vi "FormProductsTable.vi"() -> ()   [LabVIEW 2012]
uses:
  resultShow.vi
  S7Ref.vi
panel:
  in  "判定设定 2":string[][](table)
  in  "参数设定 2":string[][](table)
  in  "判定设定":string[][](table)
  in  "参数设定":string[][](table)
  in  "功能选择":T1
  in  "产品选择":bool
  in  "产品删除":bool
  in  "产品更新":bool
  in  "产品注册":bool
  in  "产品":string(combo)
  # "磨合速度"
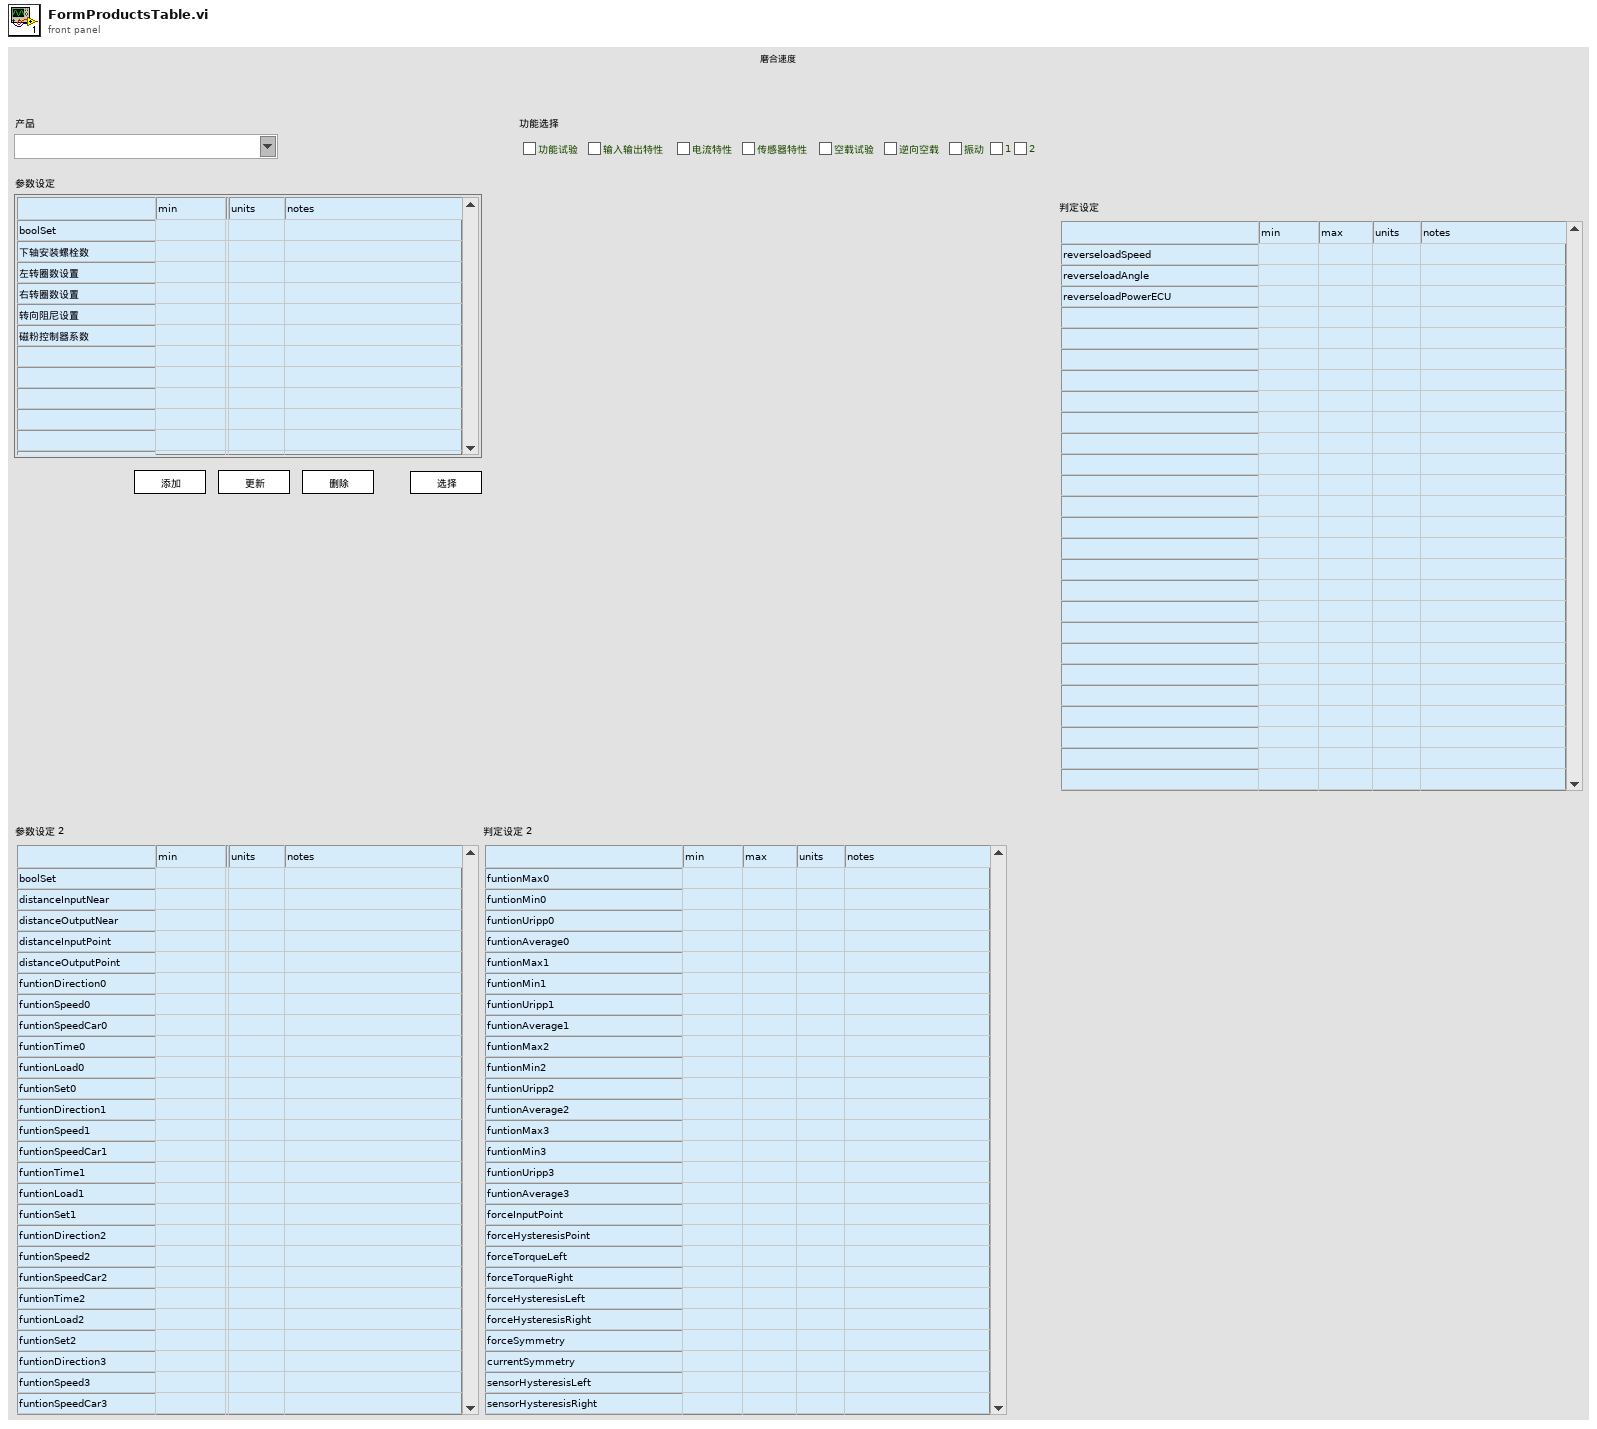
[diagram p1: front panel]
types:
  T1 = cluster{"功能试验":bool, "输入输出特性":bool, "电流特性":bool, "传感器特性":bool, "空载试验":bool, "逆向空载":bool, "振动":bool, "1":bool, "2":bool}
  T2 = enum8{"Enabled", "Disabled", "Disabled and Grayed Out"}
  T3 = enum16{"selectdata", "selectsave", "selectlist", "selectshow"}
  T4 = cluster{"userCode":string, "userName":string, "userStatus":string, "connectionMode":string, "takesTime":string, "countDone":string, "countOK":string, "countNG":string, "rigStatus":string, "productsName":string, "partCode1":string, "partCode2":string, "partCode3":string}
  T5 = cluster{"Boolean array[0]":bool, "Boolean array[1]":bool, "Boolean array[2]":bool, "Boolean array[3]":bool, "Boolean array[4]":bool, "Boolean array[5]":bool, "Boolean array[6]":bool, "Boolean array[7]":bool, "Boolean array[8]":bool}
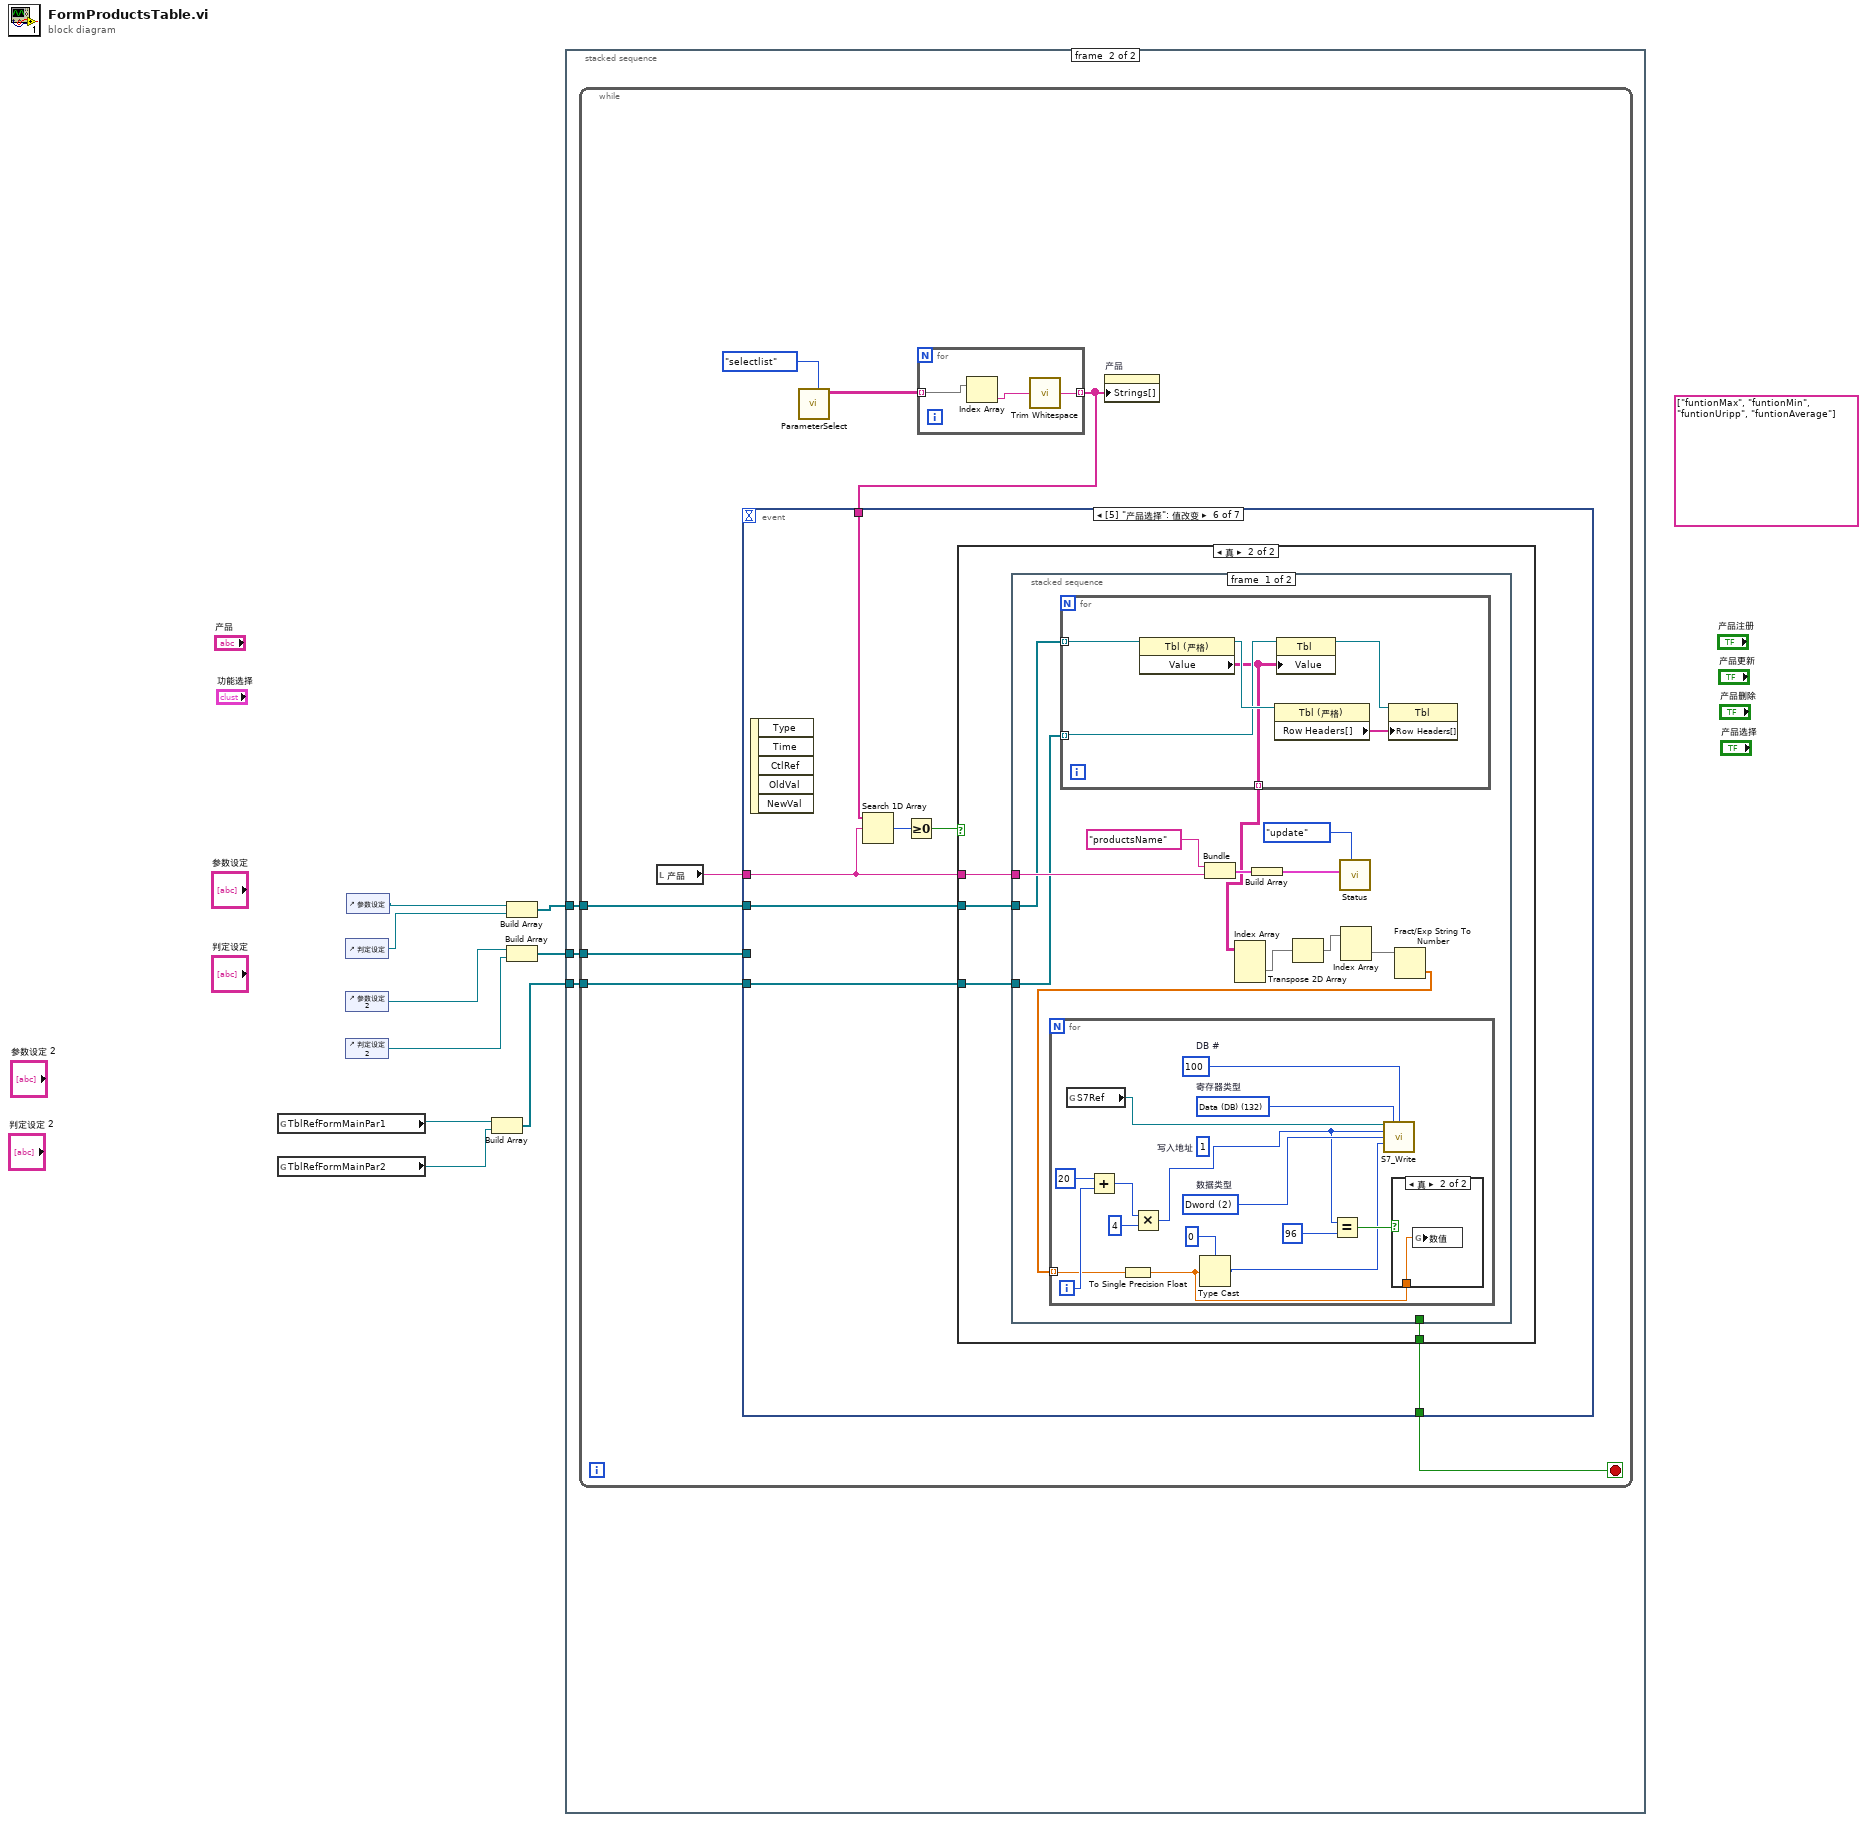
[diagram p0: block diagram]
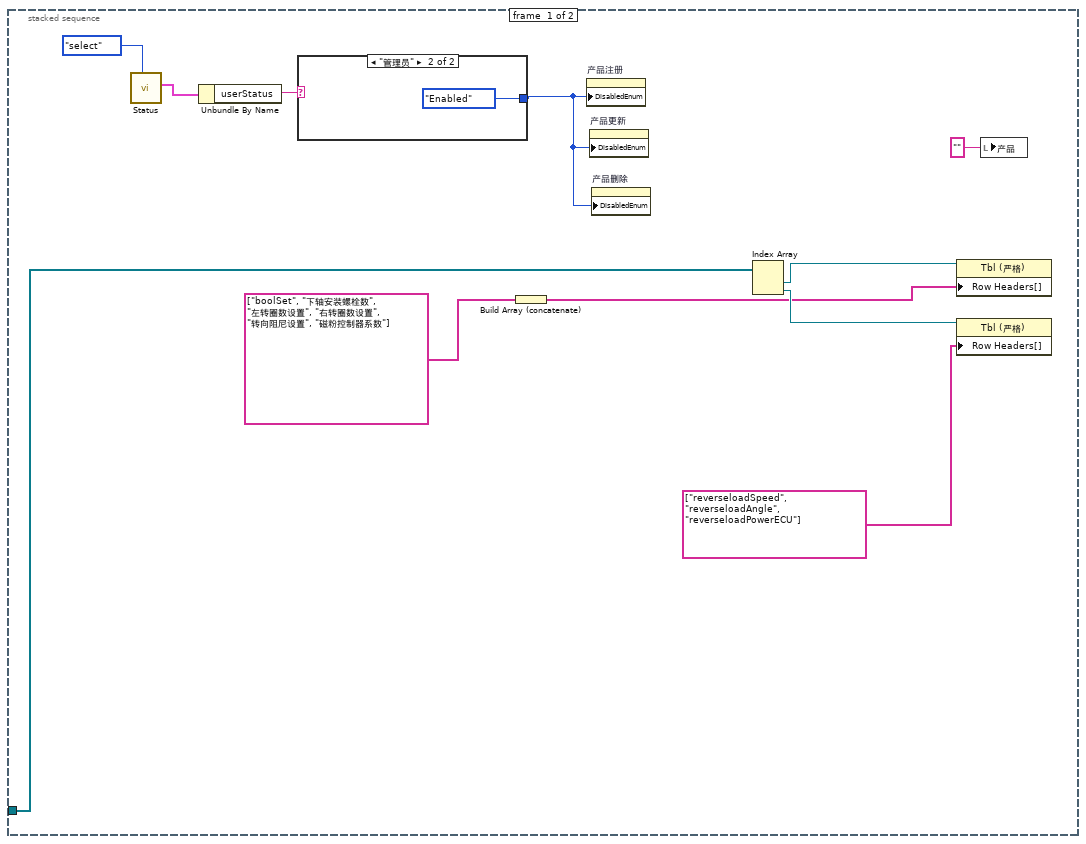
[diagram p2: hidden frame]
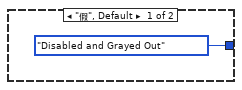
[diagram p3: hidden frame]
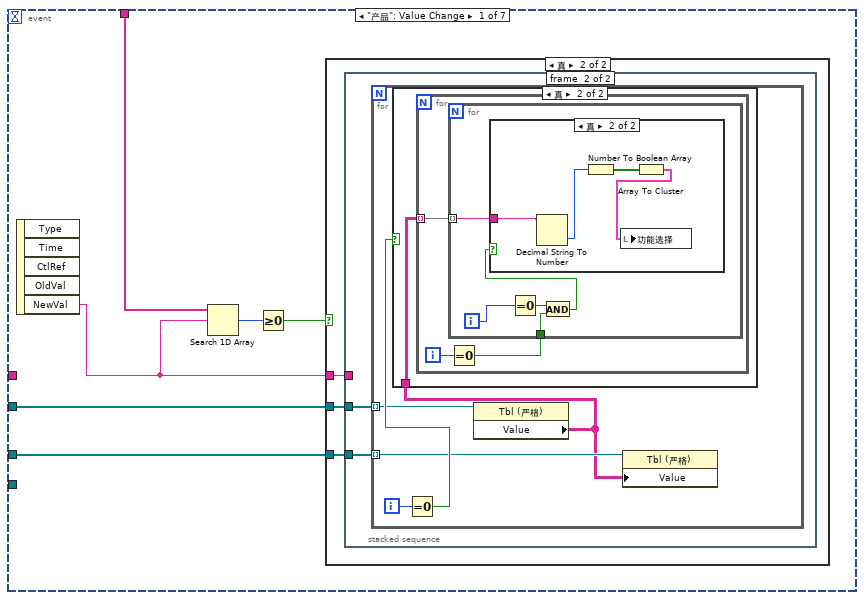
[diagram p4: hidden frame]
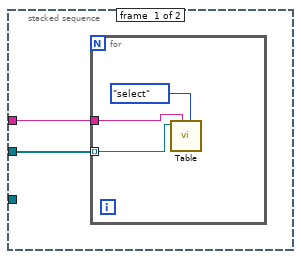
[diagram p6: hidden frame]
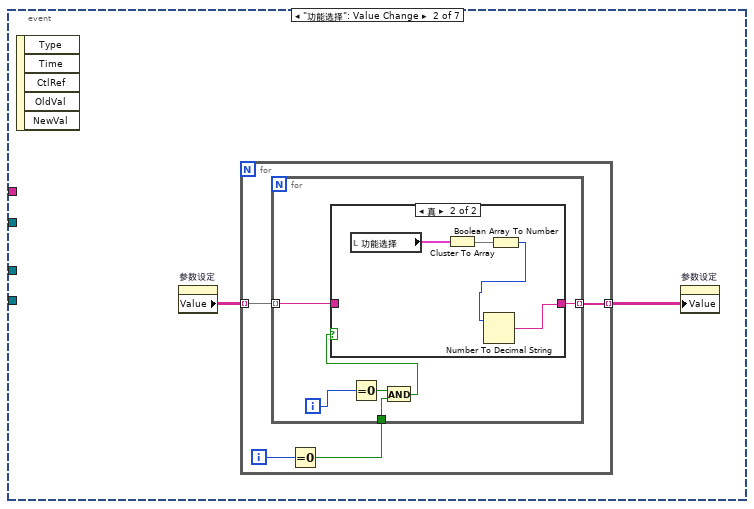
[diagram p9: hidden frame]
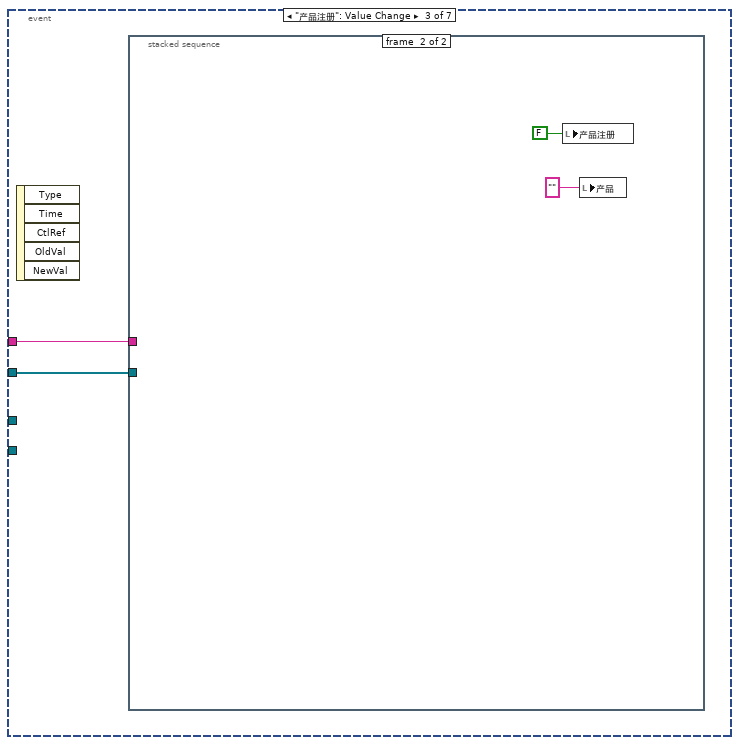
[diagram p11: hidden frame]
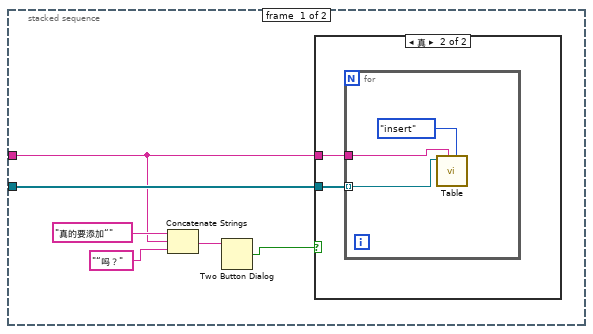
[diagram p12: hidden frame]
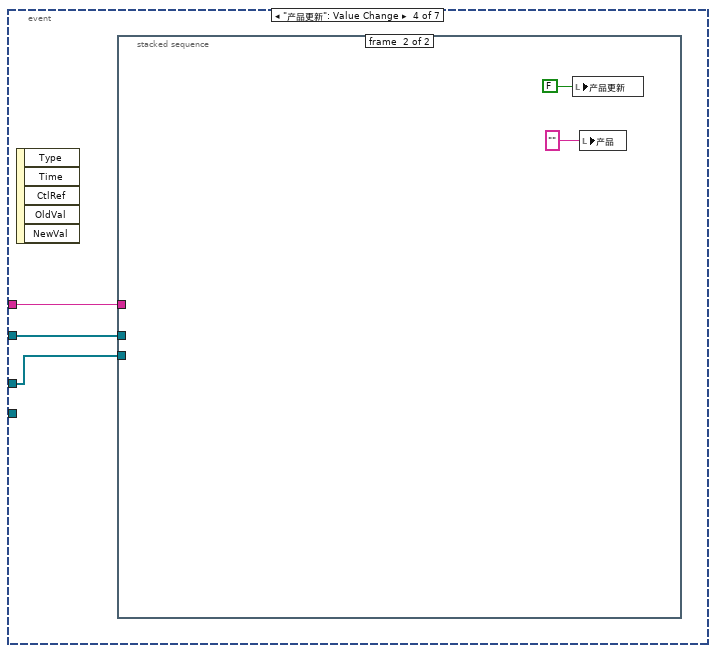
[diagram p14: hidden frame]
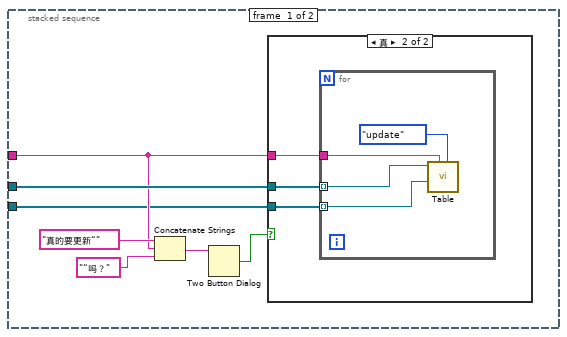
[diagram p15: hidden frame]
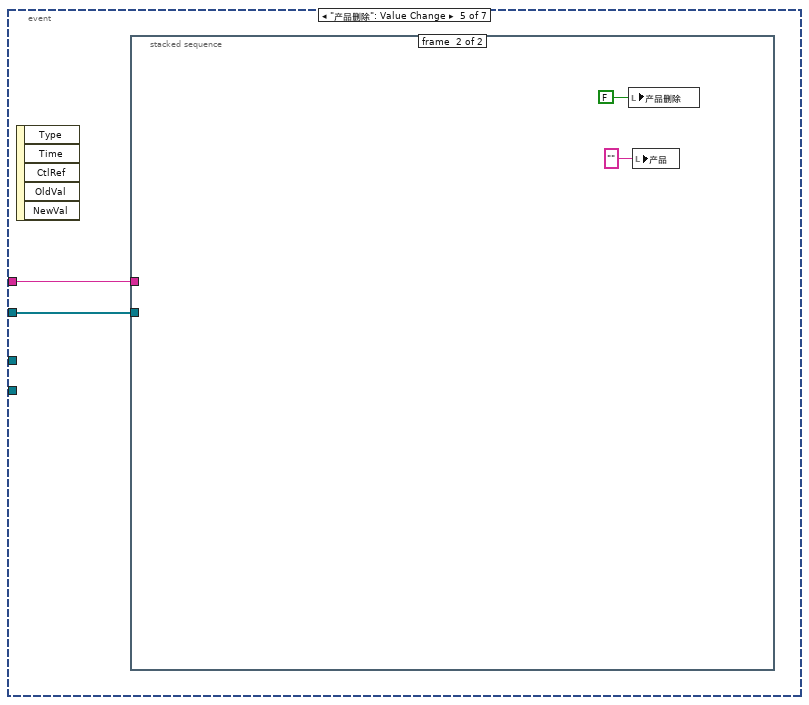
[diagram p17: hidden frame]
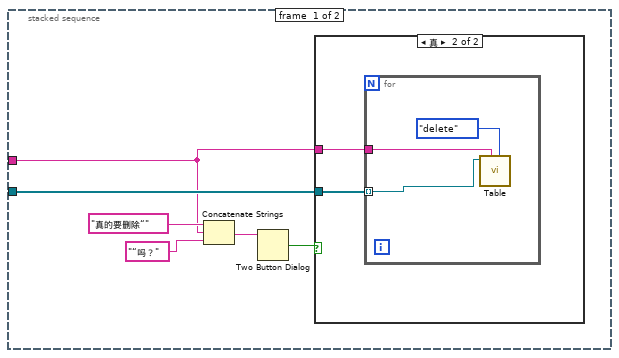
[diagram p18: hidden frame]
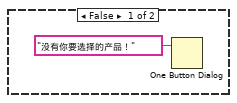
[diagram p20: hidden frame]
diagram:
  (unwired) string[] ["funtionMax", "funtionMin", "funtionUripp", "funtionAverage"] ("字符串[]")
  n1 = global read "resultShow.vi" "TblRefFormMainPar1"() -> (w5:refnum<vi>)
  n2 = global read "resultShow.vi" "TblRefFormMainPar2"() -> (w4:refnum<vi>)
  n3 = control-ref of="判定设定"() -> (w7:refnum<vi>)
  n4 = control-ref of="参数设定 2"() -> (w2:refnum<vi>)
  n5 = control-ref of="判定设定 2"() -> (w3:refnum<vi>)
  n6 = control-ref of="参数设定"() -> (w8:refnum<vi>)
  n7 = Build Array(w5, w4) -> (w6:refnum<vi>[])
  n8 = Build Array(w8, w7) -> (w9:refnum<vi>[])
  n9 = Build Array(w2, w3) -> (w1:refnum<vi>[])
  n10 = stacked-sequence {
    tunnel: w9 -> [w13 w25]
    tunnel: w6 -> [_ w24]
    tunnel: w1 -> [_ w23]
    frame #0 {
      n11 = call "Status.vi"("模式"=enum16{"select", "insert", "update", "delete"}."select") -> ("元素"=w17:T4)  [unwired: 10 in]
      n12 = Unbundle By Name(w17) -> ("userStatus"=w19:string)
      n13 = case shown="\"管理员\"" w19 {
        tunnel: [T2."Disabled and Grayed Out" ("禁用") T2."Enabled" ("禁用")] -> w16
        frame "假", Default {
        }
        frame "管理员" {
        }
      }
      n14 = Build Array (concatenate)(string[] ["boolSet", "下轴安装螺栓数", "左转圈数设置", "右转圈数设置", "转向阻尼设置", "磁粉控制器系数"] ("字符串[]")) -> (w12:string[])
      n15 = property on="产品注册" class="Bool (严格)"("DisabledEnum"=w16) -> ()  [unwired: 2 in, 2 out]
      n16 = property on="产品更新" class="Bool (严格)"("DisabledEnum"=w16) -> ()  [unwired: 2 in, 2 out]
      n17 = property on="产品删除" class="Bool (严格)"("DisabledEnum"=w16) -> ()  [unwired: 2 in, 2 out]
      n18 = Index Array(array=w13) -> (element #1=w15:refnum<vi>, element #2=w14:refnum<vi>)  [unwired: 2 in]
      n19 = property class="Tbl (严格)"(reference=w15, "Row Headers[]"=w12) -> ()  [unwired: 1 in, 2 out]
      n20 = property class="Tbl (严格)"(reference=w14, "Row Headers[]"=string[] ["reverseloadSpeed", "reverseloadAngle", "reverseloadPowerECU"] ("字符串[]")) -> ()  [unwired: 1 in, 2 out]
      n21 = local write "产品"("" ("y")) -> ()
    }
    frame #1 {
      n22 = while {
        tunnel: w25 -> [w30]
        tunnel: w24 -> [w27]
        tunnel: w23 -> [w26]
        stop <- w33 stop-if-true
        n23 = local read "产品"() -> (w32:string)
        n24 = call "ParameterSelect.vi"("模式"=T3."selectlist") -> ("dataOutAll"=w29:string[][])  [unwired: 5 in, 5 out]
        n25 = for {
          tunnel: w29 -> [w35] mode=indexing
          tunnel: [w36] -> w31 mode=indexing
          n26 = Index Array(array=w35) -> (element=w34:string)  [unwired: 1 in]
          n27 = call <vilib>:"Trim Whitespace.vi"("string"=w34) -> ("trimmed string"=w36:string)  [unwired: 1 in]
        }
        n28 = event shown="[5] \"产品选择\": 值改变" {
          selector: _ -> [_ _ _ _ _ _ _]
          dyn-events: _ -> [_ _ _ _ _ _ _]
          timeout: _ -> [_ _ _ _ _ _ _]
          tunnel: [_ _ _ _ _ w143 w189] -> w33
          tunnel: w30 -> [w42 _ w89 w105 w123 w138 _]
          tunnel: w32 -> [_ _ w88 w104 w122 w141 _]
          tunnel: w31 -> [w41 _ _ _ _ w142 _]
          tunnel: w27 -> [_ _ _ _ _ w137 _]
          tunnel: w26 -> [w37 _ _ w103 _ _ _]
          event "产品": Value Change {
            n29 = event-data() -> ("NewVal"=w39:string)  [unwired: 1 in, 4 out]
            n30 = Search 1D Array(1D array=w41, element=w39) -> (index of element=w40:i32)  [unwired: 1 in]
            n31 = Greater Or Equal To 0?(x=w40) -> (x >= 0?=w38:bool)
            n32 = case shown="真" w38 {
              tunnel: w42 -> [_ w45]
              tunnel: w39 -> [_ w44]
              tunnel: w37 -> [_ w43]
              frame False {
              }
              frame True {
                n33 = stacked-sequence {
                  tunnel: w45 -> [w47 w52]
                  tunnel: w44 -> [w46 _]
                  tunnel: w43 -> [_ w51]
                  frame #0 {
                    n34 = for {
                      tunnel: w47 -> [w50] mode=indexing
                      tunnel: w46 -> [w49]
                      n35 = call "Table.vi"("模式"=enum16{"select", "insert", "update", "delete"}."select", "productsName"=w49, "Table"=w50) -> ()  [unwired: 9 in]
                    }
                  }
                  frame #1 {
                    n36 = for {
                      tunnel: w52 -> [w55] mode=indexing
                      tunnel: w51 -> [w54] mode=indexing
                      i -> [w56]
                      n37 = Equal To 0?(x=w56) -> (x = 0?=w57:bool)
                      n38 = property on="属性节点" class="Tbl (严格)"(reference=w55) -> ("Value"=w53:string[][])  [unwired: 1 in, 2 out]
                      n39 = case shown="真" w57 {
                        tunnel: w53 -> [_ w58]
                        frame False {
                        }
                        frame True {
                          n40 = for {
                            tunnel: w58 -> [w59] mode=indexing
                            i -> [w61]
                            n41 = Equal To 0?(x=w61) -> (x = 0?=w60:bool)
                            n42 = for {
                              tunnel: w59 -> [w63] mode=indexing
                              tunnel: w60 -> [w64]
                              i -> [w65]
                              n43 = Equal To 0?(x=w65) -> (x = 0?=w66:bool)
                              n44 = And(x=w66, y=w64) -> (x .and. y?=w62:bool)
                              n45 = case shown="真" w62 {
                                tunnel: w63 -> [_ w68]
                                frame False {
                                }
                                frame True {
                                n46 = Decimal String To Number(string=w68) -> (number=w67:i32)  [unwired: 2 in, 1 out]
                                n47 = Number To Boolean Array(number=w67) -> (Boolean array=w70:bool[])
                                n48 = Array To Cluster(array=w70) -> (cluster=w69:T5)
                                n49 = local write "功能选择"(w69) -> ()
                                }
                              }
                            }
                          }
                        }
                      }
                      n50 = property on="属性节点" class="Tbl (严格)"(reference=w54, "Value"=w53) -> ()  [unwired: 1 in, 2 out]
                    }
                  }
                }
              }
            }
          }
          event "功能选择": Value Change {
            n51 = event-data() -> ()  [unwired: 1 in, 5 out]
            n52 = property on="参数设定" class="Tbl (严格)"() -> ("Value"=w72:string[][])  [unwired: 2 in, 2 out]
            n53 = for {
              tunnel: w72 -> [w76] mode=indexing
              tunnel: [w73] -> w71 mode=indexing
              i -> [w75]
              n54 = Equal To 0?(x=w75) -> (x = 0?=w74:bool)
              n55 = for {
                tunnel: w76 -> [w78] mode=indexing
                tunnel: w74 -> [w80]
                tunnel: [w79] -> w73 mode=indexing
                i -> [w81]
                n56 = Equal To 0?(x=w81) -> (x = 0?=w82:bool)
                n57 = And(x=w82, y=w80) -> (x .and. y?=w77:bool)
                n58 = case shown="真" w77 {
                  tunnel: [w83 w84] -> w79
                  tunnel: w78 -> [w83 _]
                  frame False {
                  }
                  frame True {
                    n59 = local read "功能选择"() -> (w87:T1)
                    n60 = Cluster To Array(cluster=w87) -> (array=w86:bool[])
                    n61 = Boolean Array To Number(Boolean array=w86) -> (number=w85:u32)
                    n62 = Number To Decimal String(number=w85) -> (decimal integer string=w84:string)  [unwired: 1 in]
                  }
                }
              }
            }
            n63 = property on="参数设定" class="Tbl (严格)"("Value"=w71) -> ()  [unwired: 2 in, 2 out]
          }
          event "产品注册": Value Change {
            n64 = event-data() -> ()  [unwired: 1 in, 5 out]
            n65 = stacked-sequence {
              tunnel: w89 -> [w95 _]
              tunnel: w88 -> [w90 _]
              frame #0 {
                n66 = Concatenate Strings("真的要添加“" ("消息"), w90, "“吗？" ("消息")) -> (w92:string)
                n67 = Two Button Dialog(message=w92) -> (T button?=w91:bool)  [unwired: 2 in]
                n68 = case shown="真" w91 {
                  tunnel: w95 -> [_ w97]
                  tunnel: w90 -> [_ w96]
                  frame False {
                  }
                  frame True {
                    n69 = for {
                      tunnel: w97 -> [w99] mode=indexing
                      tunnel: w96 -> [w98]
                      n70 = call "Table.vi"("模式"=enum16{"select", "insert", "update", "delete"}."insert", "productsName"=w98, "Table"=w99) -> ()  [unwired: 9 in]
                    }
                  }
                }
              }
              frame #1 {
                n71 = local write "产品注册"(FALSE ("产品注册")) -> ()
                n72 = local write "产品"("") -> ()
              }
            }
          }
          event "产品更新": Value Change {
            n73 = event-data() -> ()  [unwired: 1 in, 5 out]
            n74 = stacked-sequence {
              tunnel: w105 -> [w112 _]
              tunnel: w104 -> [w107 _]
              tunnel: w103 -> [w106 _]
              frame #0 {
                n75 = Concatenate Strings("真的要更新“" ("消息"), w107, "“吗？" ("消息")) -> (w109:string)
                n76 = Two Button Dialog(message=w109) -> (T button?=w108:bool)  [unwired: 2 in]
                n77 = case shown="真" w108 {
                  tunnel: w112 -> [_ w115]
                  tunnel: w107 -> [_ w114]
                  tunnel: w106 -> [_ w113]
                  frame False {
                  }
                  frame True {
                    n78 = for {
                      tunnel: w115 -> [w118] mode=indexing
                      tunnel: w114 -> [w117]
                      tunnel: w113 -> [w116] mode=indexing
                      n79 = call "Table.vi"("模式"=enum16{"select", "insert", "update", "delete"}."update", "productsName"=w117, "Table 2"=w116, "Table"=w118) -> ()  [unwired: 8 in]
                    }
                  }
                }
              }
              frame #1 {
                n80 = local write "产品更新"(FALSE ("产品注册")) -> ()
                n81 = local write "产品"("") -> ()
              }
            }
          }
          event "产品删除": Value Change {
            n82 = event-data() -> ()  [unwired: 1 in, 5 out]
            n83 = stacked-sequence {
              tunnel: w123 -> [w129 _]
              tunnel: w122 -> [w124 _]
              frame #0 {
                n84 = Concatenate Strings("真的要删除“" ("消息"), w124, "“吗？" ("消息")) -> (w126:string)
                n85 = Two Button Dialog(message=w126) -> (T button?=w125:bool)  [unwired: 2 in]
                n86 = case shown="真" w125 {
                  tunnel: w129 -> [_ w131]
                  tunnel: w124 -> [_ w130]
                  frame False {
                  }
                  frame True {
                    n87 = for {
                      tunnel: w131 -> [w133] mode=indexing
                      tunnel: w130 -> [w132]
                      n88 = call "Table.vi"("模式"=enum16{"select", "insert", "update", "delete"}."delete", "productsName"=w132, "Table"=w133) -> ()  [unwired: 9 in]
                    }
                  }
                }
              }
              frame #1 {
                n89 = local write "产品删除"(FALSE ("产品删除")) -> ()
                n90 = local write "产品"("" ("products_name_in")) -> ()
              }
            }
          }
          event "产品选择": Value Change {
            n91 = event-data() -> ()  [unwired: 1 in, 5 out]
            n92 = Search 1D Array(1D array=w142, element=w141) -> (index of element=w140:i32)  [unwired: 1 in]
            n93 = Greater Or Equal To 0?(x=w140) -> (x >= 0?=w139:bool)
            n94 = case shown="真" w139 {
              tunnel: [_ w148] -> w143
              tunnel: w141 -> [_ w147]
              tunnel: w138 -> [_ w146]
              tunnel: w137 -> [_ w145]
              frame False {
                n95 = One Button Dialog(message="没有你要选择的产品！" ("消息")) -> ()  [unwired: 1 in, 1 out]
              }
              frame True {
                n96 = stacked-sequence {
                  tunnel: w147 -> [w158 _]
                  tunnel: [_ TRUE ("产品删除")] -> w148
                  tunnel: w146 -> [w151 _]
                  tunnel: w145 -> [w152 _]
                  frame #0 {
                    n97 = for {
                      tunnel: w152 -> [w162] mode=indexing
                      tunnel: w151 -> [w163] mode=indexing
                      tunnel: [w161] -> w150 mode=indexing
                      n98 = property on="属性节点" class="Tbl (严格)"(reference=w163) -> (reference out=w165:refnum<vi>, "Value"=w161:string[][])  [unwired: 1 in, 1 out]
                      n99 = property on="属性节点" class="Tbl (严格)"(reference=w165) -> ("Row Headers[]"=w164:string[])  [unwired: 1 in, 2 out]
                      n100 = property on="属性节点" class="Tbl"(reference=w162, "Value"=w161) -> (reference out=w166:refnum<vi>)  [unwired: 1 in, 1 out]
                      n101 = property on="属性节点" class="Tbl"(reference=w166, "Row Headers[]"=w164) -> ()  [unwired: 1 in, 2 out]
                    }
                    n102 = Bundle("name"="productsName", "产品"=w158) -> (w157:cluster{"name":string, "产品":string})  [unwired: 1 in]
                    n103 = Index Array(array=w150) -> (element=w149:string[][])  [unwired: 3 in]
                    n104 = Build Array(w157) -> (w156:cluster{"name":string, "产品":string}[])
                    n105 = Transpose 2D Array(2D array=w149) -> (transposed array=w153:string[][])
                    n106 = call "Status.vi"("模式"=enum16{"select", "insert", "update", "delete"}."update", "nameData"=w156) -> ()  [unwired: 9 in, 1 out]
                    n107 = Index Array(array=w153) -> (element=w155:string[])  [unwired: 2 in]
                    n108 = Fract/Exp String To Number(string=w155) -> (number=w154:dbl[])  [unwired: 3 in, 1 out]
                    n109 = for {
                      tunnel: w154 -> [w172] mode=indexing
                      i -> [w175]
                      w180 = u16 2 items=["byte", "word", "Dword"]  # 数据类型
                      (unwired) u32 1  # 写入地址
                      w179 = u16 100  # DB #
                      w181 = u8 132 items=["I/O (P)"=128, "Input (I)"=129, "Output (Q)"=130, "Bit Memory (M)"=131, "Data (DB)"=132, "Instance Data (DI)"=133, "Local Data (L)"=134, "Predecessor Local Data (VL)"=135]  # 寄存器类型
                      n110 = global read "S7Ref.vi" "S7Ref"() -> (w177:refnum<k5>)
                      n111 = Add(x=20 ("y"), y=w175) -> (x+y=w174:i32)
                      n112 = To Single Precision Float(number=w172) -> (single precision float=w167:sgl)
                      n113 = Multiply(x=w174, y=4) -> (x*y=w171:i32)
                      n114 = Type Cast(type=u32 0, x=w167) -> (*(type *) &x=w168:u32)
                      n115 = Equal?(x=w171, y=96) -> (x = y?=w169:bool)
                      n116 = call "S7_Write.vi"("TCP"=w177, "寄存器类型"=w181, "DB #"=w179, "写入地址"=w171, "数据类型"=w180, "写入数据"=w168) -> ()  [unwired: 7 in, 3 out]
                      n117 = case shown="真" w169 {
                        tunnel: w167 -> [_ w182]
                        frame False {
                        }
                        frame True {
                          n118 = global write "resultShow.vi" "数值"(w182) -> ()
                        }
                      }
                    }
                  }
                  frame #1 {
                    n119 = case shown="真" TRUE {
                      frame False {
                      }
                      frame True {
                        n120 = property on="窗格" class="Pane"() -> ("OwningVI"=w188:refnum<vi>)  [unwired: 2 in, 2 out]
                        n121 = property on="属性节点" class="VI"(reference=w188) -> ("Name"=w187:string)  [unwired: 1 in, 2 out]
                        n122 = call "CloseVI.vi"("名称或相对路径"=w187) -> ()  [unwired: 10 in, 1 out]
                      }
                    }
                    n123 = local write "产品选择"(FALSE ("产品删除")) -> ()
                    n124 = local write "产品"("") -> ()
                  }
                }
              }
            }
          }
          event Panel Close? {
            w189 = TRUE
            n125 = event-data() -> ()  [unwired: 1 in, 3 out]
            n126 = Not(x=w189) -> (.not. x?=w190:bool)
            n127 = event-data("Discard?"=w190) -> ()  [unwired: 1 in, 1 out]
          }
        }
        n128 = property on="产品" class="CmbBox"("Strings[]"=w31) -> ()  [unwired: 2 in, 2 out]
      }
    }
  }
